vi "dfd_Quantizer (I32).vi"(5 "q_mode":T1=enum."Truncation" caption="round mode", 7 "LSB pos":i32, 11 "I32 in":i32[](array[numeric])) -> (3 "I32 out":i32[](array[numeric]))   [LabVIEW 2017, in "NI_DigFilter_FXP.lvlib"]
uses:
  <vilib>/addons/Digital Filter Design/NI_DigFilter_FXP.lvlib
  <vilib>/addons/Digital Filter Design/_Objects.llb/DFD Round-off Mode.ctl
  <vilib>/addons/Digital Filter Design/NI_DigFilterLicensed.lvlib
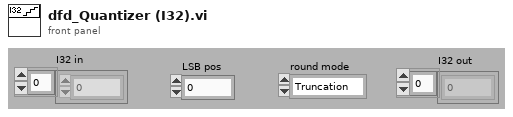
[diagram p1: front panel]
types:
  T1 = typedef "NI_DigFilterLicensed.lvlib/DFD Round-off Mode.ctl" = enum16{"Nearest", "Truncation"}
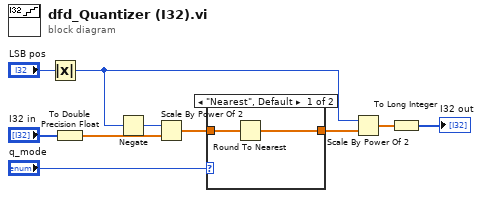
[diagram p0: block diagram]
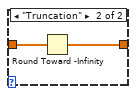
[diagram p2: hidden frame]
diagram:
  n1 = Absolute Value(x="LSB pos") -> (abs(x)=w8:i32)
  n2 = To Double Precision Float(number="I32 in") -> (double precision float=w6:dbl[])
  n3 = Negate(x=w8) -> (-x=w7:i32)
  n4 = Scale By Power Of 2(n=w7, x=w6) -> (x*2^n=w4:dbl[])
  n5 = case shown="\"Nearest\", Default" "q_mode" {
    tunnel: w4 -> [w12 w14]
    tunnel: [w11 w13] -> w3
    frame "Nearest", Default {
      n6 = Round To Nearest(number=w12) -> (nearest integer value=w11:dbl[])
    }
    frame "Truncation" {
      n7 = Round Toward -Infinity(1:w14) -> (0:w13:dbl[])
    }
  }
  n8 = Scale By Power Of 2(n=w8, x=w3) -> (x*2^n=w2:dbl[])
  n9 = To Long Integer(number=w2) -> (32bit integer=→"I32 out":i32[])
